vi "getStreamPath.vi"(8 "error in (no error)":errorcluster, 11 "AnalogOutput.lvclass in":refnum<class "AnalogOutput.lvclass">) -> (0 "error out":errorcluster, 2 "streamPath":path, 3 "AnalogOutput.lvclass out":refnum<class "AnalogOutput.lvclass">)   [LabVIEW 2011, in "Hardware.lvlib" / "Channels.lvlib" / "AnalogOutput.lvclass"]
uses:
  AnalogOutput.lvclass
  AnalogOutput.lvclass/AnalogOutput.ctl
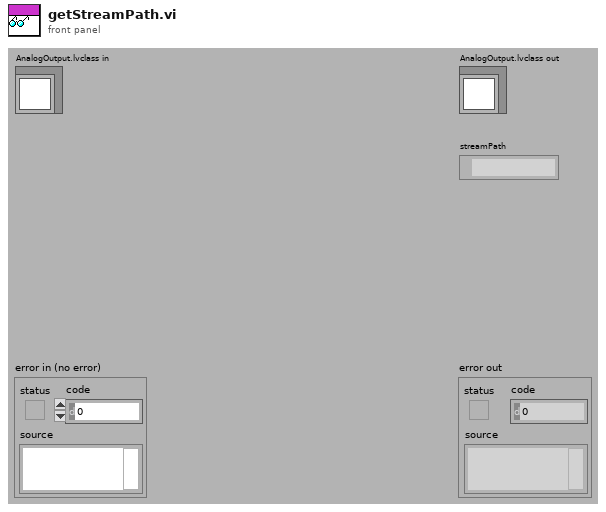
[diagram p1: front panel]
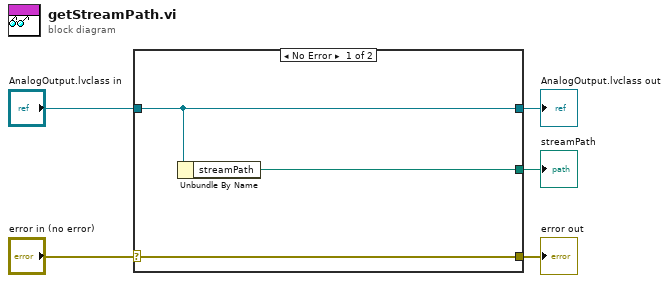
[diagram p0: block diagram]
diagram:
  n1 = case shown="No Error" "error in (no error)" {
    selector: "error in (no error)" -> [w8 w9]
    tunnel: [w8 w9] -> w4
    tunnel: [w7 w10] -> w2
    tunnel: "AnalogOutput.lvclass in" -> [w7 w10]
    tunnel: [w6 _] -> w1
    frame No Error {
      n2 = Unbundle By Name(w7) -> ("streamPath"=w6:path)
    }
    frame Error {
    }
  }
  "error out" <- w4
  "AnalogOutput.lvclass out" <- w2
  "streamPath" <- w1
